vi "Check Input Data to Array.vi"(8 "error in (no error)":errorcluster, 11 "String Array/ String":variant) -> (0 "error out":errorcluster, 3 "ColumnsNameList":string[](array[string]))   [LabVIEW 2021, in "DataBase_SQL.lvclass"]
uses:
  <userlib>/John_Lib/DataBase/DataBase_SQL/DataBase_SQL.lvclass
  <userlib>/John_Lib/DataBase/DataBase_SQL/DataBase_SQL.lvclass/DataBase_SQL.ctl
  <vilib>/Utility/Data Type/NI_Data Type.lvlib
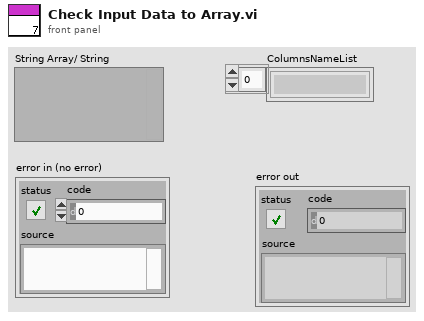
[diagram p1: front panel]
types:
  T1 = typedef "NI_Data Type.lvlib/Data Type.ctl" = enum8{"Invalid Type", "Void", "I8", "I16", "I32", "I64", "U8", "U16", "U32", "U64", "Single Float", "Double Float", "Extended Float", "Single Complex", "Double Complex", "Extended Complex", "Enum U8", "Enum U16", "Enum U32", "Enum U64", "Single Float With Unit", "Double Float With Unit", "Extended Float With Unit", "Single Complex with Unit", "Double Complex with Unit", "Extended Complex with Unit", "Boolean", "String", "Path", "Picture", "Tag", "Array", "Cluster", "Variant", "LV Variant", "Waveform", "Timestamp", "Digital Waveform", "Digital Data", "ExpressData", "Refnum", "External Data", "VI", "Poly VI", "LabVIEW Class Instance", "Fixed Point", "Set Collection", "Map Collection"}
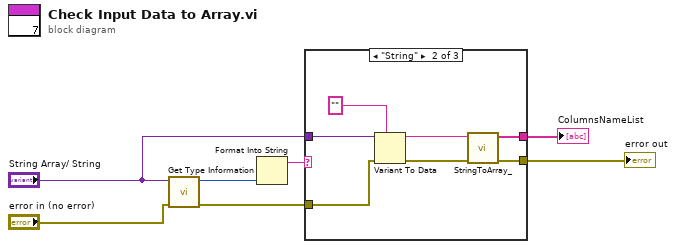
[diagram p0: block diagram]
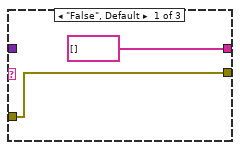
[diagram p2: hidden frame]
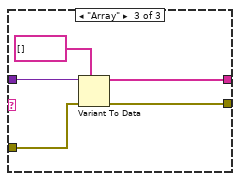
[diagram p3: hidden frame]
diagram:
  n1 = call <vilib>:"Get Type Information.vi"("error in (no error)"="error in (no error)", "variant"="String Array/ String") -> ("error out"=w2:errorcluster, "type"=w7:T1)  [unwired: 5 in, 3 out]
  n2 = Format Into String(w7) -> (resulting string=w6:string)  [unwired: 3 in, 1 out]
  n3 = case shown="\"String\"" w6 {
    tunnel: "String Array/ String" -> [_ w15 w20]
    tunnel: [string[] [] ("Array") w12 w18] -> w4
    tunnel: w2 -> [w8 w11 w17]
    tunnel: [w8 w10 w16] -> w1
    frame "False", Default {
    }
    frame "String" {
      n4 = Variant To Data(error in=w11, type="" ("State Queue"), Variant=w15) -> (data=w13:string, error out=w10:errorcluster)
      n5 = call <userlib>:"StringToArray_.vi"("State Queue"=w13) -> ("Array"=w12:string[])  [unwired: 7 in, 3 out]
    }
    frame "Array" {
      n6 = Variant To Data(error in=w17, type=string[] [] ("ColumnsNameList"), Variant=w20) -> (data=w18:string[], error out=w16:errorcluster)
    }
  }
  "ColumnsNameList" <- w4
  "error out" <- w1
